vi "Unpack Notification Msg.vi"(11 "Notification Msg":refnum<class "Notification Msg.lvclass">) -> (1 "Publication Time":timestamp, 2 "Value":variant, 3 "Datum Name":string)   [LabVIEW 2020, in "ActorMessageTransport.lvlib" / "Notification Msg.lvclass"]
doc: "Unpacks the data from a fulfilled Notification Msg.\n\n*** DO NOT OVERRIDE THIS METHOD ***\nDynamic Dispatch added to this method for backwards compatibility in MVA Framework. DD will be removed in a future release."
uses:
  <vilib>/gpm_packages/@cs/transport/Source/Concrete/ActorMessageTransport/Notification Msg/Notification Msg.lvclass
  <vilib>/gpm_packages/@cs/transport/Source/Concrete/ActorMessageTransport/Notification Msg/Notification Msg.lvclass/Notification Msg.ctl
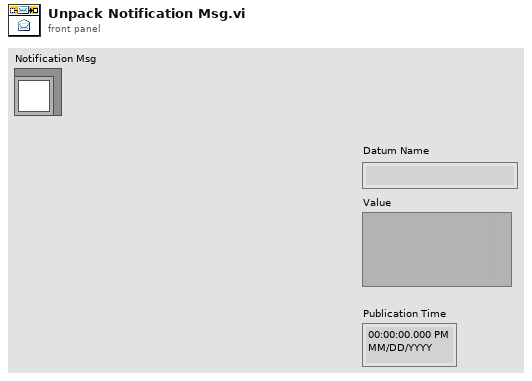
[diagram p1: front panel]
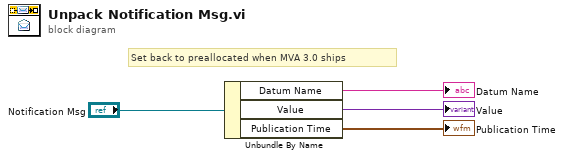
[diagram p0: block diagram]
diagram:
  # "Set back to preallocated when MVA 3.0 ships"
  n1 = Unbundle By Name("Notification Msg") -> ("Datum Name"=→"Datum Name":string, "Value"=→"Value":variant, "Publication Time"=→"Publication Time":timestamp)
